vi "lua execution control.vi"() -> (0 "error out":errorcluster)   [LabVIEW 2020]
uses:
  Instance           5 29Saved   lua execution control .vi
  Instance          11 29Saved   lua execution control .vi
panel:
  in  "LUA Script":string="-- Use USER_RAM0_U16 (register 46180) to determine which control loop to run\n\nlocal ramval = 0\n\nMB.W(46180, 0, ramval)\n\nlocal loop0 = 0\n\nlocal loop1 = 1\n\nlocal loop2 = 2\n\n-- Setup an interval to control loop execution speed. Update every second\n\nLJ.IntervalConfig(0,1000)\n\nwhile true do\n\n  if LJ.CheckInterval(0) then\n\n    ramval = MB.R(46180, 0)\n\n    if ramval == loop0 then\n\n      print(\"using loop0\")\n\n    end\n\n    if ramval == loop1 then\n\n      print(\"using loop1\")\n\n    end\n\n    if ramval == loop2 then\n\n      print(\"using loop2\")\n\n    end\n\n  end\n\nend\n\u0000" caption="Result"
  out "Lua Message":string
  out "Lua Debug Num Bytes":dbl format="%.2f"
  in  "Interval (ms)":u32=1000
  out "Script Length":i32
  out "Error String":string="No Error"
  out "ConnectionType Out":i32
  out "DeviceType Out":i32
  in  "Identifier":string="LJM_idANY"
  in  "ConnectionType":string="LJM_ctANY"
  in  "DeviceType":string="LJM_dtANY"
  # "This example demonstrates how a lua script can be created,loaded, and controlled in LabVIEW using LJM"
  # "Match the interval to the lua script interval. Be mindful that the timing of the lua script may vary slightly from the timing in LabVIEW"
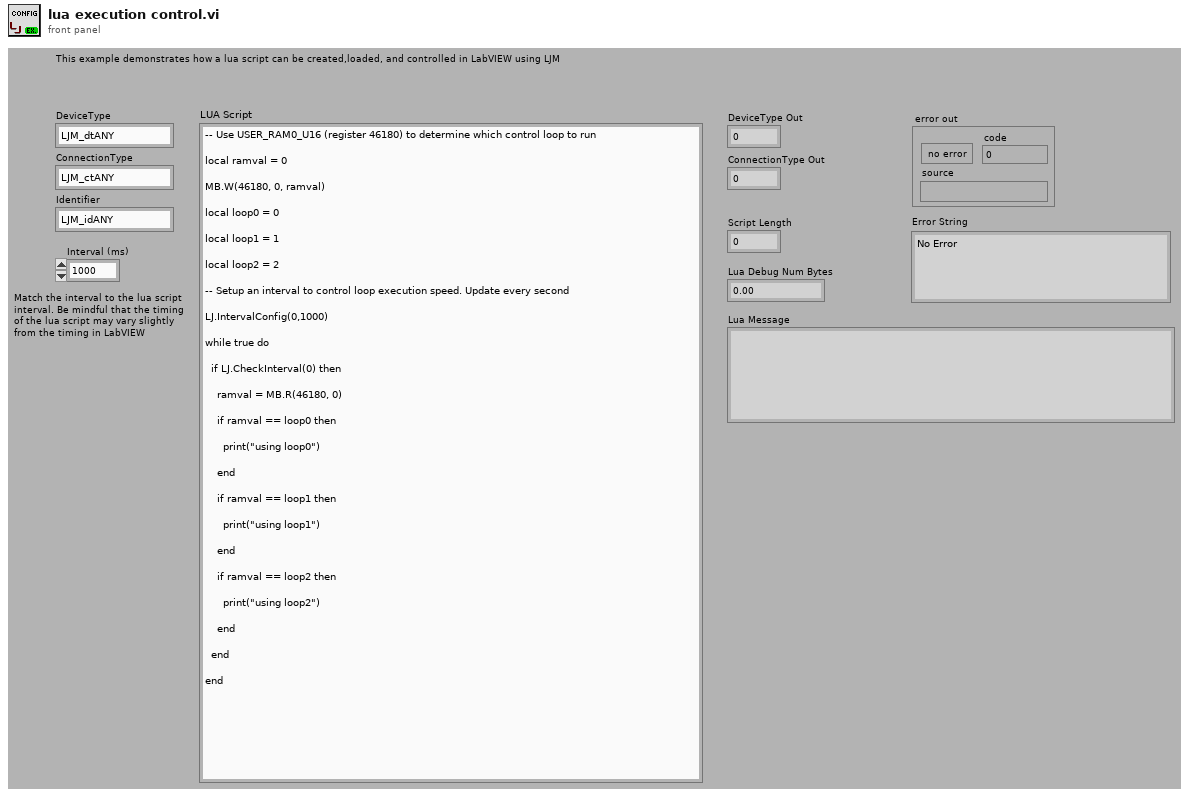
[diagram p1: front panel]
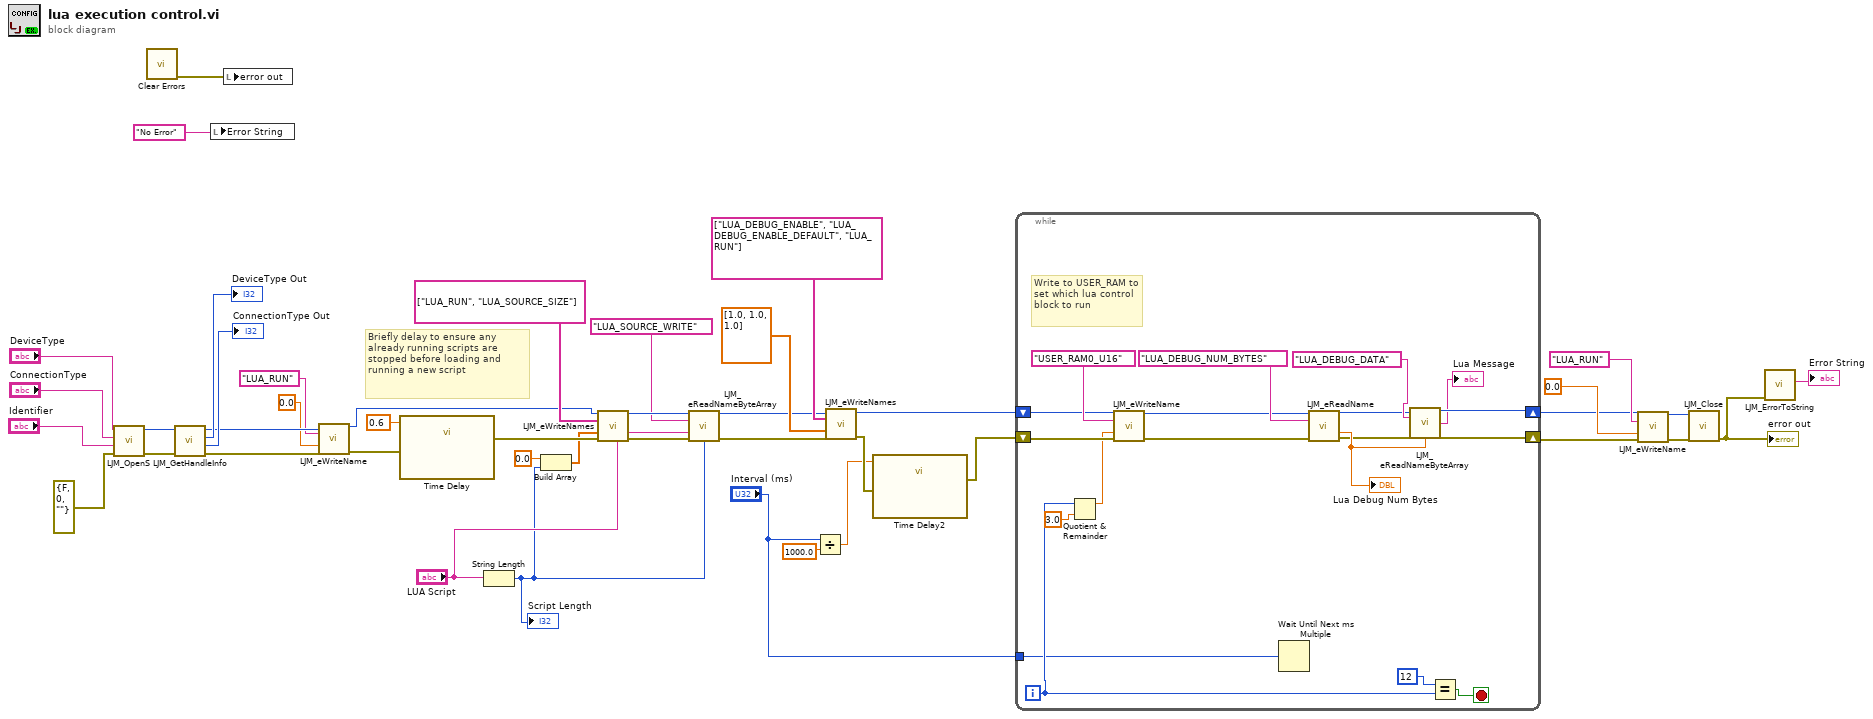
[diagram p0: block diagram]
diagram:
  # "Briefly delay to ensure any already running scripts are stopped before loading and running a new script"
  n1 = call "LJM_OpenS.vi"("error in"=errorcluster {"status"=FALSE, "code"=0, "source"=""} ("error in (no error)"), "Identifier"="Identifier", "ConnectionType"="ConnectionType", "DeviceType"="DeviceType") -> ("error out"=w43:errorcluster, "Handle"=w42:i32)  [unwired: 6 in]
  n2 = call <vilib>:"Clear Errors.vi"() -> ("error out"=w2:errorcluster)  [unwired: 6 in, 1 out]
  n3 = call "LJM_GetHandleInfo.vi"("error in"=w43, "Handle In"=w42) -> ("error out"=w32:errorcluster, "ConnectionType"=→"ConnectionType Out":i32, "DeviceType"=→"DeviceType Out":i32, "Handle Out"=w33:i32)  [unwired: 2 in, 4 out]
  n4 = local write "Error String"("No Error" ("Error String")) -> ()
  n5 = local write "error out"(w2) -> ()
  n6 = call "LJM_eWriteName.vi"("Handle In"=w33, "Name"="LUA_RUN", "Value"=0.0, "error in"=w32) -> ("Handle Out"=w27:i32, "error out"=w7:errorcluster)  [unwired: 10 in]
  n7 = call "Time Delay"("error in (no error)"=w7, "Delay Time (s)"=0.6) -> ("error out"=w28:errorcluster)  [unwired: 9 in]
  n8 = String Length(string="LUA Script") -> (length=w6:i32)
  "Script Length" <- w6
  n9 = Build Array(0.0 ("element"), w6) -> (w23:dbl[])
  n10 = call "LJM_eWriteNames.vi"("Handle In"=w27, "aNames"=string[] ["LUA_RUN", "LUA_SOURCE_SIZE"], "aValuesIn"=w23, "error in"=w28) -> ("Handle Out"=w20:i32, "error out"=w21:errorcluster)  [unwired: 9 in, 1 out]
  n11 = call "LJM_eReadNameByteArray.vi"("Handle In"=w20, "Name"="LUA_SOURCE_WRITE", 9:"LUA Script", "error in"=w21, "NumBytes"=w6) -> ("Handle Out"=w17:i32, "error out"=w18:errorcluster)  [unwired: 7 in, 2 out]
  n12 = Divide(x="Interval (ms)", y=1000.0) -> (x/y=w4:dbl)
  n13 = call "LJM_eWriteNames.vi"("Handle In"=w17, "aNames"=string[] ["LUA_DEBUG_ENABLE", "LUA_DEBUG_ENABLE_DEFAULT", "LUA_RUN"], "aValuesIn"=dbl[] [1.0, 1.0, 1.0], "error in"=w18) -> ("Handle Out"=w22:i32, "error out"=w10:errorcluster)  [unwired: 9 in, 1 out]
  n14 = call "Time Delay2"("error in (no error)"=w10, "Delay Time (s)"=w4) -> ("error out"=w9:errorcluster)  [unwired: 9 in]
  n15 = while {
    shift-right: [w47] -> w14
    shift-left: w9 -> [w59]
    shift-right: [w48] -> w13
    shift-left: w22 -> [w60]
    tunnel: "Interval (ms)" -> [w45]
    i -> [w53]
    stop <- w63 stop-if-true
    # "Write to USER_RAM to set which lua control block to run"
    n16 = Quotient & Remainder(x=w53, y=3.0) -> (x-y*floor(x/y)=w55:dbl)  [unwired: 1 out]
    n17 = call "LJM_eWriteName.vi"("Handle In"=w60, "Name"="USER_RAM0_U16", "Value"=w55, "error in"=w59) -> ("Handle Out"=w56:i32, "error out"=w57:errorcluster)  [unwired: 10 in]
    n18 = Wait Until Next ms Multiple(millisecond multiple=w45) -> ()  [unwired: 1 out]
    n19 = call "LJM_eReadName.vi"("Handle In"=w56, "Name"="LUA_DEBUG_NUM_BYTES", "error in"=w57) -> ("Handle Out"=w49:i32, "Value"=w52:dbl, "error out"=w51:errorcluster)  [unwired: 10 in]
    "Lua Debug Num Bytes" <- w52
    n20 = call "LJM_eReadNameByteArray.vi"("Handle In"=w49, "Name"="LUA_DEBUG_DATA", "error in"=w51, "NumBytes"=w52) -> ("Handle Out"=w48:i32, "aBytes"=→"Lua Message":string, "error out"=w47:errorcluster)  [unwired: 8 in, 1 out]
    n21 = Equal?(x=12, y=w53) -> (x = y?=w63:bool)
  }
  n22 = call "LJM_eWriteName.vi"("Handle In"=w13, "Name"="LUA_RUN", "Value"=0.0, "error in"=w14) -> ("Handle Out"=w12:i32, "error out"=w11:errorcluster)  [unwired: 10 in]
  n23 = call "LJM_Close.vi"("error in"=w11, "Handle"=w12) -> ("error out"=w36:errorcluster)  [unwired: 9 in]
  "error out" <- w36
  n24 = call "LJM_ErrorToString.vi"("error in"=w36) -> ("String"=→"Error String":string)  [unwired: 10 in]
